vi "Actor Core.vi"(8 "error in":errorcluster, 11 "TRExperimentsRaw in":refnum<class "Samples.lvclass">) -> (0 "error out":errorcluster, 3 "Actor out":refnum<class "Actor.lvclass">)   [LabVIEW 2020, in "Forms.lvlib" / "Samples.lvclass"]
doc: "The user interface for this panel.\n\n----\nPlease see the following web address for additional documentation and tutorial information:\nhttp://www.mooregoodideas.com/mgi-panel-manager/\n\nAuthor: Derek Trepanier\n\nCopyright (c) 2018, Moore Good Ideas, Inc.\n\nAll rights reserved.\n\nRedistribution and use in source and binary forms, with or without modification, are permitted provided that the following conditions are met:\n\n * Redistributions of source code must retain the above copyright notice, this list of conditions and the following disclaimer.\n * Redistributions in binary form must reproduce the above copyright notice, this list of conditions and the following disclaimer in the documentation and/or other materials provided with the distribution.\n * Neither the name of Moore Good Ideas, Inc. nor the names of its contributors may be used to endorse or promote products derived from this software without specific prior written permission.\n\nTHIS SOFTWARE IS PROVIDED BY THE COPYRIGHT HOLDERS AND CONTRIBUTORS \"AS IS\" AND ANY EXPRESS OR IMPLIED WARRANTIES, INCLUDING, BUT NOT LIMITED TO, THE IMPLIED WARRANTIES OF MERCHANTABILITY AND FITNESS FOR A PARTICULAR PURPOSE ARE DISCLAIMED. IN NO EVENT SHALL THE COPYRIGHT OWNER OR CONTRIBUTORS BE LIABLE FOR ANY DIRECT, INDIRECT, INCIDENTAL, SPECIAL, EXEMPLARY, OR CONSEQUENTIAL DAMAGES (INCLUDING, BUT NOT LIMITED TO, PROCUREMENT OF SUBSTITUTE GOODS OR SERVICES; LOSS OF USE, DATA, OR PROFITS; OR BUSINESS INTERRUPTION) HOWEVER CAUSED AND ON ANY THEORY OF LIABILITY, WHETHER IN CONTRACT, STRICT LIABILITY, OR TORT (INCLUDING NEGLIGENCE OR OTHERWISE) ARISING IN ANY WAY OUT OF THE USE OF THIS SOFTWARE, EVEN IF ADVISED OF THE POSSIBILITY OF SUCH DAMAGE."
uses:
  Samples.lvclass
  C:/Users/User/Desktop/Raman Program/Database OOP/source/Forms AF/Forms Controller/Form Controller/Panel Form Controller.lvclass
  <vilib>/ActorFramework/Actor/Actor.lvclass
  Users/Users/Users.lvclass
  Sample Chemical Formula/Sample Chemical Formula.lvclass
  Forms Controller/Form Controller/Panel Form Controller.lvclass/Panel Form Controller.ctl
  Database OOP/Column Libraries/Basic Fields/Field Configurations/Field Configuration Class/Field Configuration.lvclass
  C:/Users/User/Desktop/Raman Program/Database OOP/source/Database OOP/Column Libraries/Field Interfaces/Field Configuration Interface Class/Field Configuration.lvclass
  Forms Controller/Open Form Button/Open Form Button.lvclass
  C:/Users/User/Desktop/Raman Program/Database OOP/source/Database OOP/Button Libraries/Button Interface Class/Button Interface.lvclass
  Database OOP/Column Libraries/Basic Field Constructors/Numeric Field.vi
  Database OOP/Column Libraries/Basic Field Constructors/Text Field.vi
  Database OOP/Column Libraries/Basic Field Constructors/FK Ring Field.vi
  Forms Controller/Form Window/Form Window.lvclass
  Database OOP/Table Libraries/Basic Form/Basic Form.lvclass
  Database OOP/Column Libraries/Basic Field Constructors.lvlib
  Forms Controller/Form Controller/Panel Form Controller.lvclass
panel:
  in  "Add Formula":bool
  in  "Add User":bool
  in  "Chemical Formula":u16(ring)
  in  "User":u16(ring)
  in  "Doping Density (%)":dbl
  in  "Display Name":string
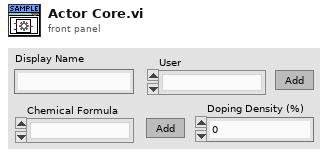
[diagram p1: front panel]
types:
  T1 = typedef "Panel Form Controller.lvlib/Builder Cluster.ctl" = cluster{"VI Ctrl Array":refnum<vi>[], "Form":refnum<class "Basic Form.lvclass">, "Open Form Button":refnum<class "Open Form Button.lvclass">}
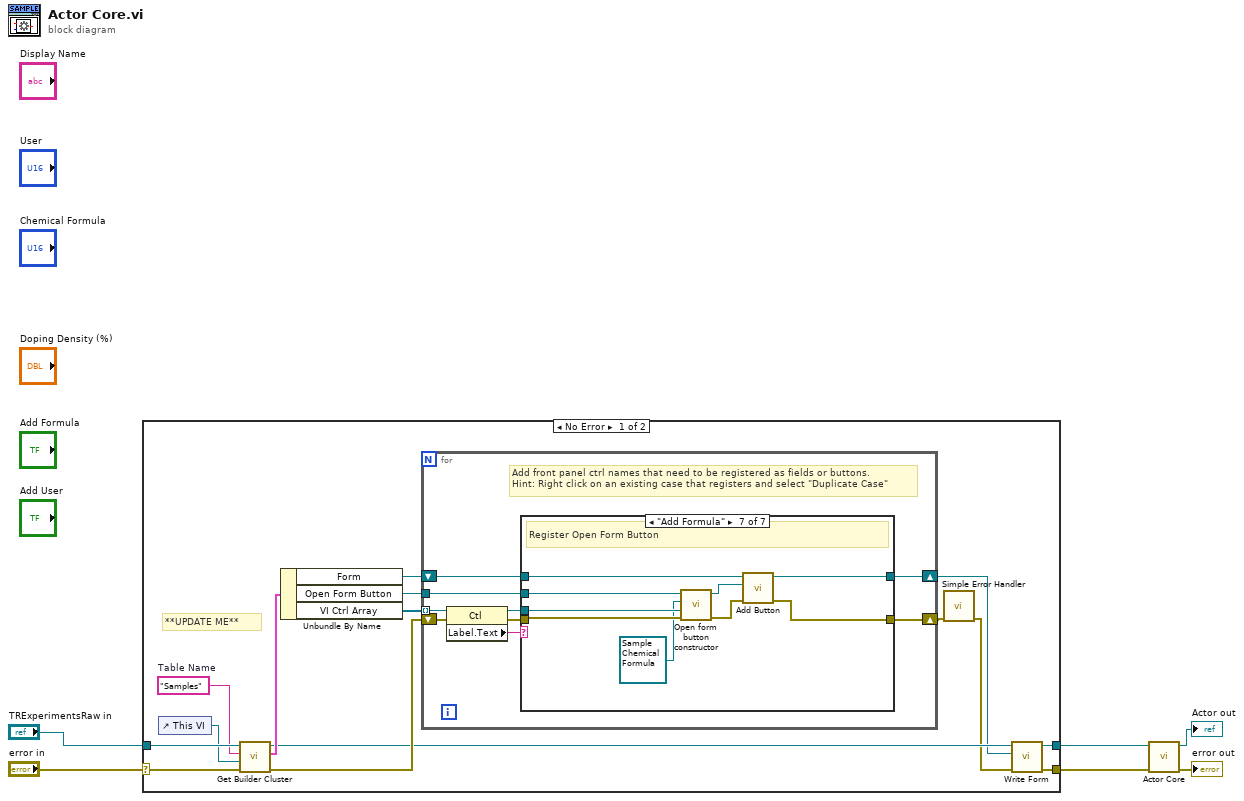
[diagram p0: block diagram]
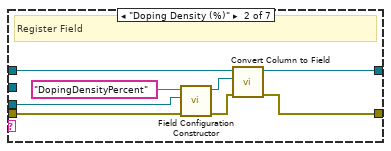
[diagram p3: hidden frame]
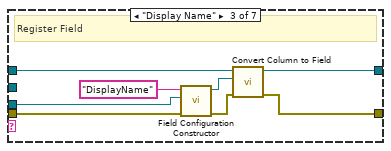
[diagram p4: hidden frame]
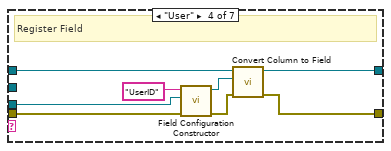
[diagram p5: hidden frame]
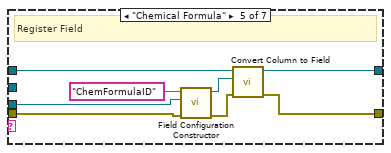
[diagram p6: hidden frame]
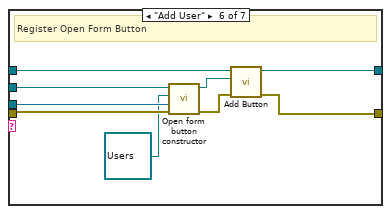
[diagram p7: hidden frame]
diagram:
  n1 = case shown="No Error" "error in" {
    selector: "error in" -> [w16 w84]
    tunnel: "TRExperimentsRaw in" -> [w20 w83]
    tunnel: [w9 w84] -> w2
    tunnel: [w10 w83] -> w1
    frame No Error {
      w7 = "Samples"  # Table Name
      # "**UPDATE ME**"
      n2 = control-ref of="This VI"() -> (w8:refnum<vi>)
      n3 = call "Get Builder Cluster.vi"("error in (no error)"=w16, "VI Refnum"=w8, "Table Name"=w7, "Panel Form Controller in"=w20) -> ("error out"=w18:errorcluster, "Builder Cluster"=w17:T1, "Panel Form Controller out"=w13:refnum<class "Samples.lvclass">)  [unwired: 5 in]
      n4 = Unbundle By Name(w17) -> ("Form"=w19:refnum<class "Basic Form.lvclass">, "Open Form Button"=w14:refnum<class "Open Form Button.lvclass">, "VI Ctrl Array"=w15:refnum<vi>[])
      n5 = for {
        tunnel: w15 -> [w30] mode=indexing
        shift-right: [w23] -> w11
        shift-left: w19 -> [w24]
        shift-right: [w28] -> w21
        shift-left: w18 -> [w27]
        tunnel: w14 -> [w22]
        # "Add front panel ctrl names that need to be registered as fields or buttons.\nHint: Right click on an existing case that registers and select \"Duplicate Case\""
        n6 = property class="Ctl"(reference=w30, error in=w27) -> (reference out=w29:refnum<vi>, error out=w26:errorcluster, "Label.Text"=w25:string)
        n7 = case shown="\"Add Formula\"" w25 {
          tunnel: w29 -> [_ w35 w43 w52 w60 w67 w76]
          tunnel: w24 -> [w32 w40 w48 w56 w64 w73 w82]
          tunnel: [w32 w38 w46 w54 w62 w72 w81] -> w23
          tunnel: [w31 w39 w47 w55 w63 w71 w80] -> w28
          tunnel: w26 -> [w31 w34 w42 w51 w59 w66 w75]
          tunnel: w22 -> [_ _ _ _ _ w68 w77]
          frame "", Default {
            # "Not Registered"
          }
          frame "Doping Density (%)" {
            # "Register Field"
            n8 = call-poly "Field Configuration Constructor.vi"("error in"=w34, "Ctl Refnum"=w35, "Column Name"="DopingDensityPercent" ("Column")) -> ("error out"=w37:errorcluster, "Field Configuration"=w33:refnum<class "Field Configuration.lvclass">)  [unwired: 7 in]
            n9 = call "Convert Column to Field.vi"("error in (no error)"=w37, "Field Configuration"=w33, "Basic Form in"=w40) -> ("error out"=w39:errorcluster, "Basic Form out"=w38:refnum<class "Basic Form.lvclass">)  [unwired: 7 in]
          }
          frame "Display Name" {
            # "Register Field"
            n10 = call-poly "Field Configuration Constructor.vi"("error in"=w42, "Ctl Refnum"=w43, "Column Name"="DisplayName" ("Column")) -> ("error out"=w45:errorcluster, "Field Configuration"=w41:refnum<class "Field Configuration.lvclass">)  [unwired: 7 in]
            n11 = call "Convert Column to Field.vi"("error in (no error)"=w45, "Field Configuration"=w41, "Basic Form in"=w48) -> ("error out"=w47:errorcluster, "Basic Form out"=w46:refnum<class "Basic Form.lvclass">)  [unwired: 7 in]
          }
          frame "User" {
            # "Register Field"
            n12 = call-poly "Field Configuration Constructor.vi"("error in"=w51, "Ctl Refnum"=w52, "Column Name"="UserID" ("Column")) -> ("error out"=w53:errorcluster, "Field Configuration"=w50:refnum<class "Field Configuration.lvclass">)  [unwired: 7 in]
            n13 = call "Convert Column to Field.vi"("error in (no error)"=w53, "Field Configuration"=w50, "Basic Form in"=w56) -> ("error out"=w55:errorcluster, "Basic Form out"=w54:refnum<class "Basic Form.lvclass">)  [unwired: 7 in]
          }
          frame "Chemical Formula" {
            # "Register Field"
            n14 = call-poly "Field Configuration Constructor.vi"("error in"=w59, "Ctl Refnum"=w60, "Column Name"="ChemFormulaID" ("Column")) -> ("error out"=w61:errorcluster, "Field Configuration"=w58:refnum<class "Field Configuration.lvclass">)  [unwired: 7 in]
            n15 = call "Convert Column to Field.vi"("error in (no error)"=w61, "Field Configuration"=w58, "Basic Form in"=w64) -> ("error out"=w63:errorcluster, "Basic Form out"=w62:refnum<class "Basic Form.lvclass">)  [unwired: 7 in]
          }
          frame "Add User" {
            # "Register Open Form Button"
            n16 = call "Open form button constructor.vi"("error in (no error)"=w66, "Ctl Refnum"=w67, "Panel Form"=refnum<class "Users.lvclass"> refnum ("Forms.lvlib:Users.lvclass"), "Open Form Button in"=w68) -> ("error out"=w69:errorcluster, "Open Form Button out"=w70:refnum<class "Open Form Button.lvclass">)  [unwired: 6 in]
            n17 = call "Add Button.vi"("error in (no error)"=w69, "Button"=w70, "Basic Form in"=w73) -> ("error out"=w71:errorcluster, "Basic Form out"=w72:refnum<class "Basic Form.lvclass">)  [unwired: 7 in]
          }
          frame "Add Formula" {
            # "Register Open Form Button"
            n18 = call "Open form button constructor.vi"("error in (no error)"=w75, "Ctl Refnum"=w76, "Panel Form"=refnum<class "Sample Chemical Formula.lvclass"> refnum ("Forms.lvlib:Sample Chemical Formula.lvclass"), "Open Form Button in"=w77) -> ("error out"=w78:errorcluster, "Open Form Button out"=w79:refnum<class "Open Form Button.lvclass">)  [unwired: 6 in]
            n19 = call "Add Button.vi"("error in (no error)"=w78, "Button"=w79, "Basic Form in"=w82) -> ("error out"=w80:errorcluster, "Basic Form out"=w81:refnum<class "Basic Form.lvclass">)  [unwired: 7 in]
          }
        }
      }
      n20 = call <vilib>:"Simple Error Handler.vi"("error in (no error)"=w21) -> ("error out"=w12:errorcluster)  [unwired: 4 in, 4 out]
      n21 = call "Write Form.vi"("error in (no error)"=w12, "Form.lvlib:Basic Form.lvclass"=w11, "Panel Form Controller in"=w13) -> ("error out"=w9:errorcluster, "Panel Form Controller out"=w10:refnum<class "Samples.lvclass">)  [unwired: 7 in]
    }
    frame Error {
    }
  }
  n22 = call-parent "Actor Core.vi"("error in"=w2, "Form Window in"=w1) -> ("error out"=→"error out":errorcluster, "Actor out"=→"Actor out":refnum<class "Actor.lvclass">)  [unwired: 8 in]
